vi "DPT Worksheet DOE Audit.vi"(0 "2015?":bool, 1 "Add?":bool, 5 "DOE Data":T1={"Technician"="", "Date"="", "Model"="", "Serial"="", "Total Dry Time(m)"=0.0, "Bone Dry Wt"=0.0, "Initial Wt"=0.0, "Final Wt"=0.0, "Initial Ret"=0.0, "Final Ret"=0.0, "Elect Energy Used"=0.0, "Gas Meter Temp"=0.0, "Gas Meter Pres"=0.0, "Gas Volume"=0.0, "Barometer Temp"=70.0, "Barometer Pres"=0.0, "Gas Corr Fact"=0.0, "Cor Gas Vol"=0.0, "Gas Heat Val"=0.0, "Gas Energy BTU"=0.0, "Gas Energy kwh 4%"=0.0, "Elect Energy kwh 4%"=0.0, "Total  Energy 4%"=0.0, "Gas Vol Init"=0.0, "Gas Vol Fin"=0.0, "Start Time(s)"=0.0, "End Time(s)"=0.0, "Elect Energy Start"=0.0, "Elect Energy End"=0.0, "Per Cycle Efficency"=0.0, "Annual Consumption"=0.0, "Load Cycles"="", "Ambinet Temp"="", "Ambinet RH"="", "Per Cycle Off Mode/Standby Power"=0.0, "Total Energy (Gas + Elect)"=0.0, "Combined Energy Factor"=0.0, "Off Mode Power"=0.0, "Exhaust"="", "Washer Water Temperature ( 60 ± 5°F )"="", "Supply Voltage"="", "Reference Temperature (F)"="", "Reference Pressure (psi)"="", "Standby Power"=0.0}, 12 "Write Form":bool) -> (6 "DOE Data Out":T1={"Technician"="", "Date"="", "Model"="", "Serial"="", "Total Dry Time(m)"=0.0, "Bone Dry Wt"=0.0, "Initial Wt"=0.0, "Final Wt"=0.0, "Initial Ret"=0.0, "Final Ret"=0.0, "Elect Energy Used"=0.0, "Gas Meter Temp"=0.0, "Gas Meter Pres"=0.0, "Gas Volume"=0.0, "Barometer Temp"=70.0, "Barometer Pres"=0.0, "Gas Corr Fact"=0.0, "Cor Gas Vol"=0.0, "Gas Heat Val"=0.0, "Gas Energy BTU"=0.0, "Gas Energy kwh 4%"=0.0, "Elect Energy kwh 4%"=0.0, "Total  Energy 4%"=0.0, "Gas Vol Init"=0.0, "Gas Vol Fin"=0.0, "Start Time(s)"=0.0, "End Time(s)"=0.0, "Elect Energy Start"=0.0, "Elect Energy End"=0.0, "Per Cycle Efficency"=0.0, "Annual Consumption"=0.0, "Load Cycles"="", "Ambinet Temp"="", "Ambinet RH"="", "Per Cycle Off Mode/Standby Power"=0.0, "Total Energy (Gas + Elect)"=0.0, "Combined Energy Factor"=0.0, "Off Mode Power"=0.0, "Exhaust"="", "Washer Water Temperature ( 60 ± 5°F )"="", "Supply Voltage"="", "Reference Temperature (F)"="", "Reference Pressure (psi)"="", "Standby Power"=0.0}, 10 "2015 array":string[][](array[string]), 15 "String":string)   [LabVIEW 2016, in "File Setup.lvlib"]
uses:
  File Setup.lvlib
  Type Definition/DPT Audit Data.ctl
panel:
  # "Add Water Hardness\nand panel"
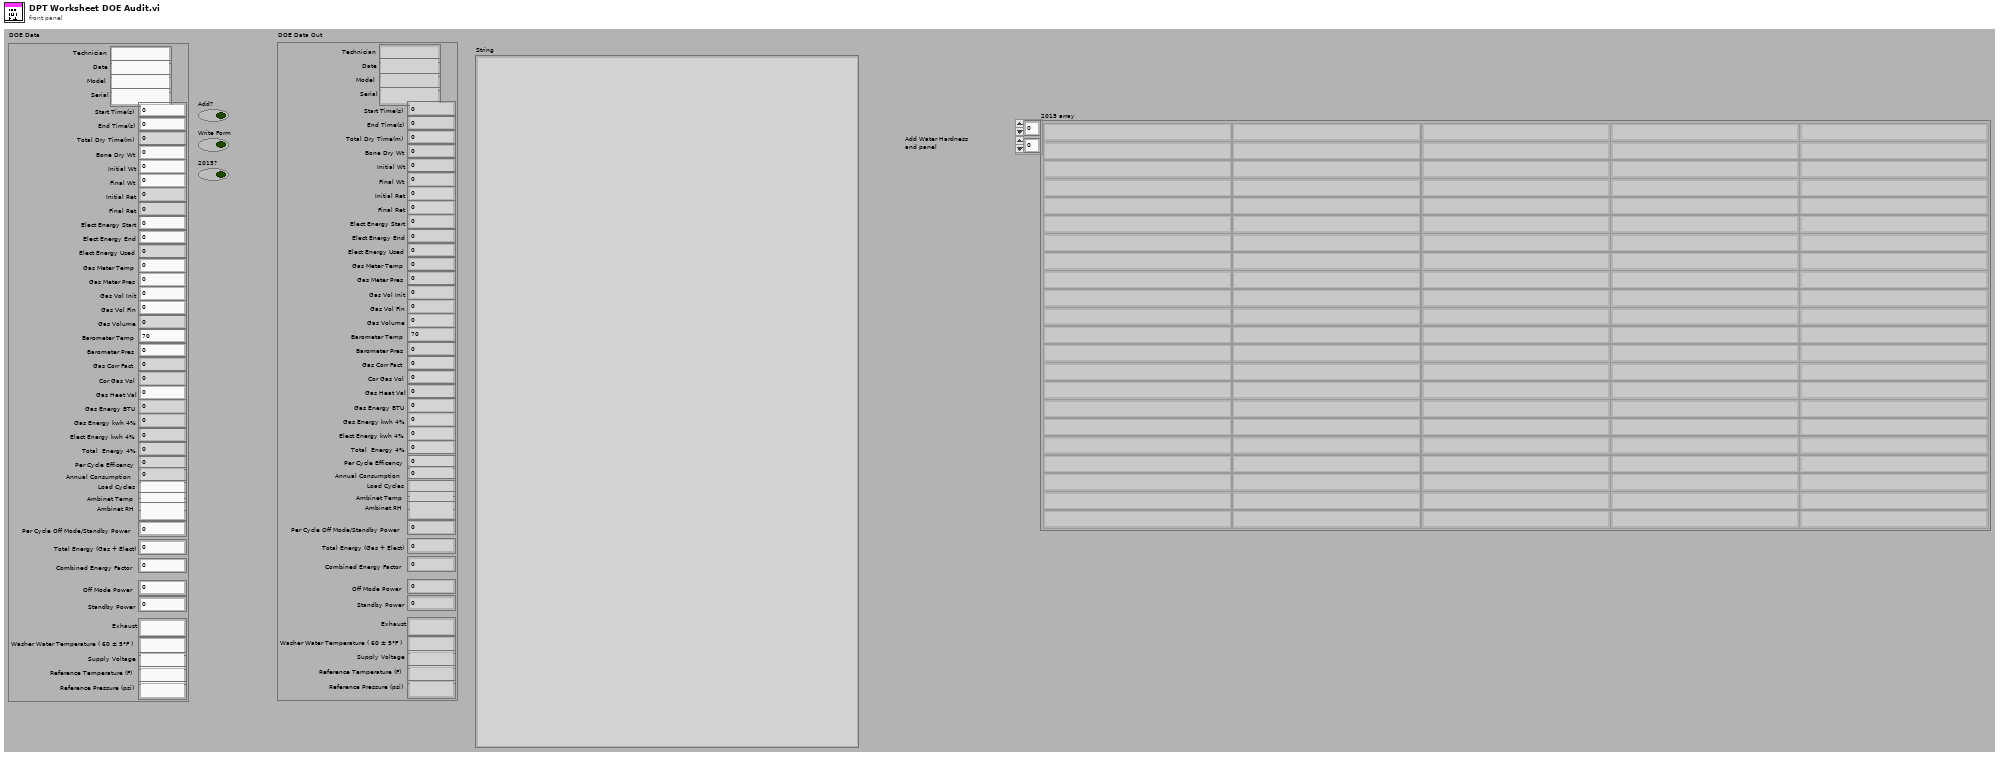
[diagram p1: front panel]
types:
  T1 = typedef "File Setup.lvlib/DPT Audit Data.ctl" = cluster{"Technician":string, "Date":string, "Model":string, "Serial":string, "Total Dry Time(m)":dbl, "Bone Dry Wt":dbl, "Initial Wt":dbl, "Final Wt":dbl, "Initial Ret":dbl, "Final Ret":dbl, "Elect Energy Used":dbl, "Gas Meter Temp":dbl, "Gas Meter Pres":dbl, "Gas Volume":dbl, "Barometer Temp":dbl, "Barometer Pres":dbl, "Gas Corr Fact":dbl, "Cor Gas Vol":dbl, "Gas Heat Val":dbl, "Gas Energy BTU":dbl, "Gas Energy kwh 4%":dbl, "Elect Energy kwh 4%":dbl, "Total  Energy 4%":dbl, "Gas Vol Init":dbl, "Gas Vol Fin":dbl, "Start Time(s)":dbl, "End Time(s)":dbl, "Elect Energy Start":dbl, "Elect Energy End":dbl, "Per Cycle Efficency":dbl, "Annual Consumption":dbl, "Load Cycles":string, "Ambinet Temp":string, "Ambinet RH":string, "Per Cycle Off Mode/Standby Power":dbl, "Total Energy (Gas + Elect)":dbl, "Combined Energy Factor":dbl, "Off Mode Power":dbl, "Exhaust":string, "Washer Water Temperature ( 60 ± 5°F )":string, "Supply Voltage":string, "Reference Temperature (F)":string, "Reference Pressure (psi)":string, "Standby Power":dbl}
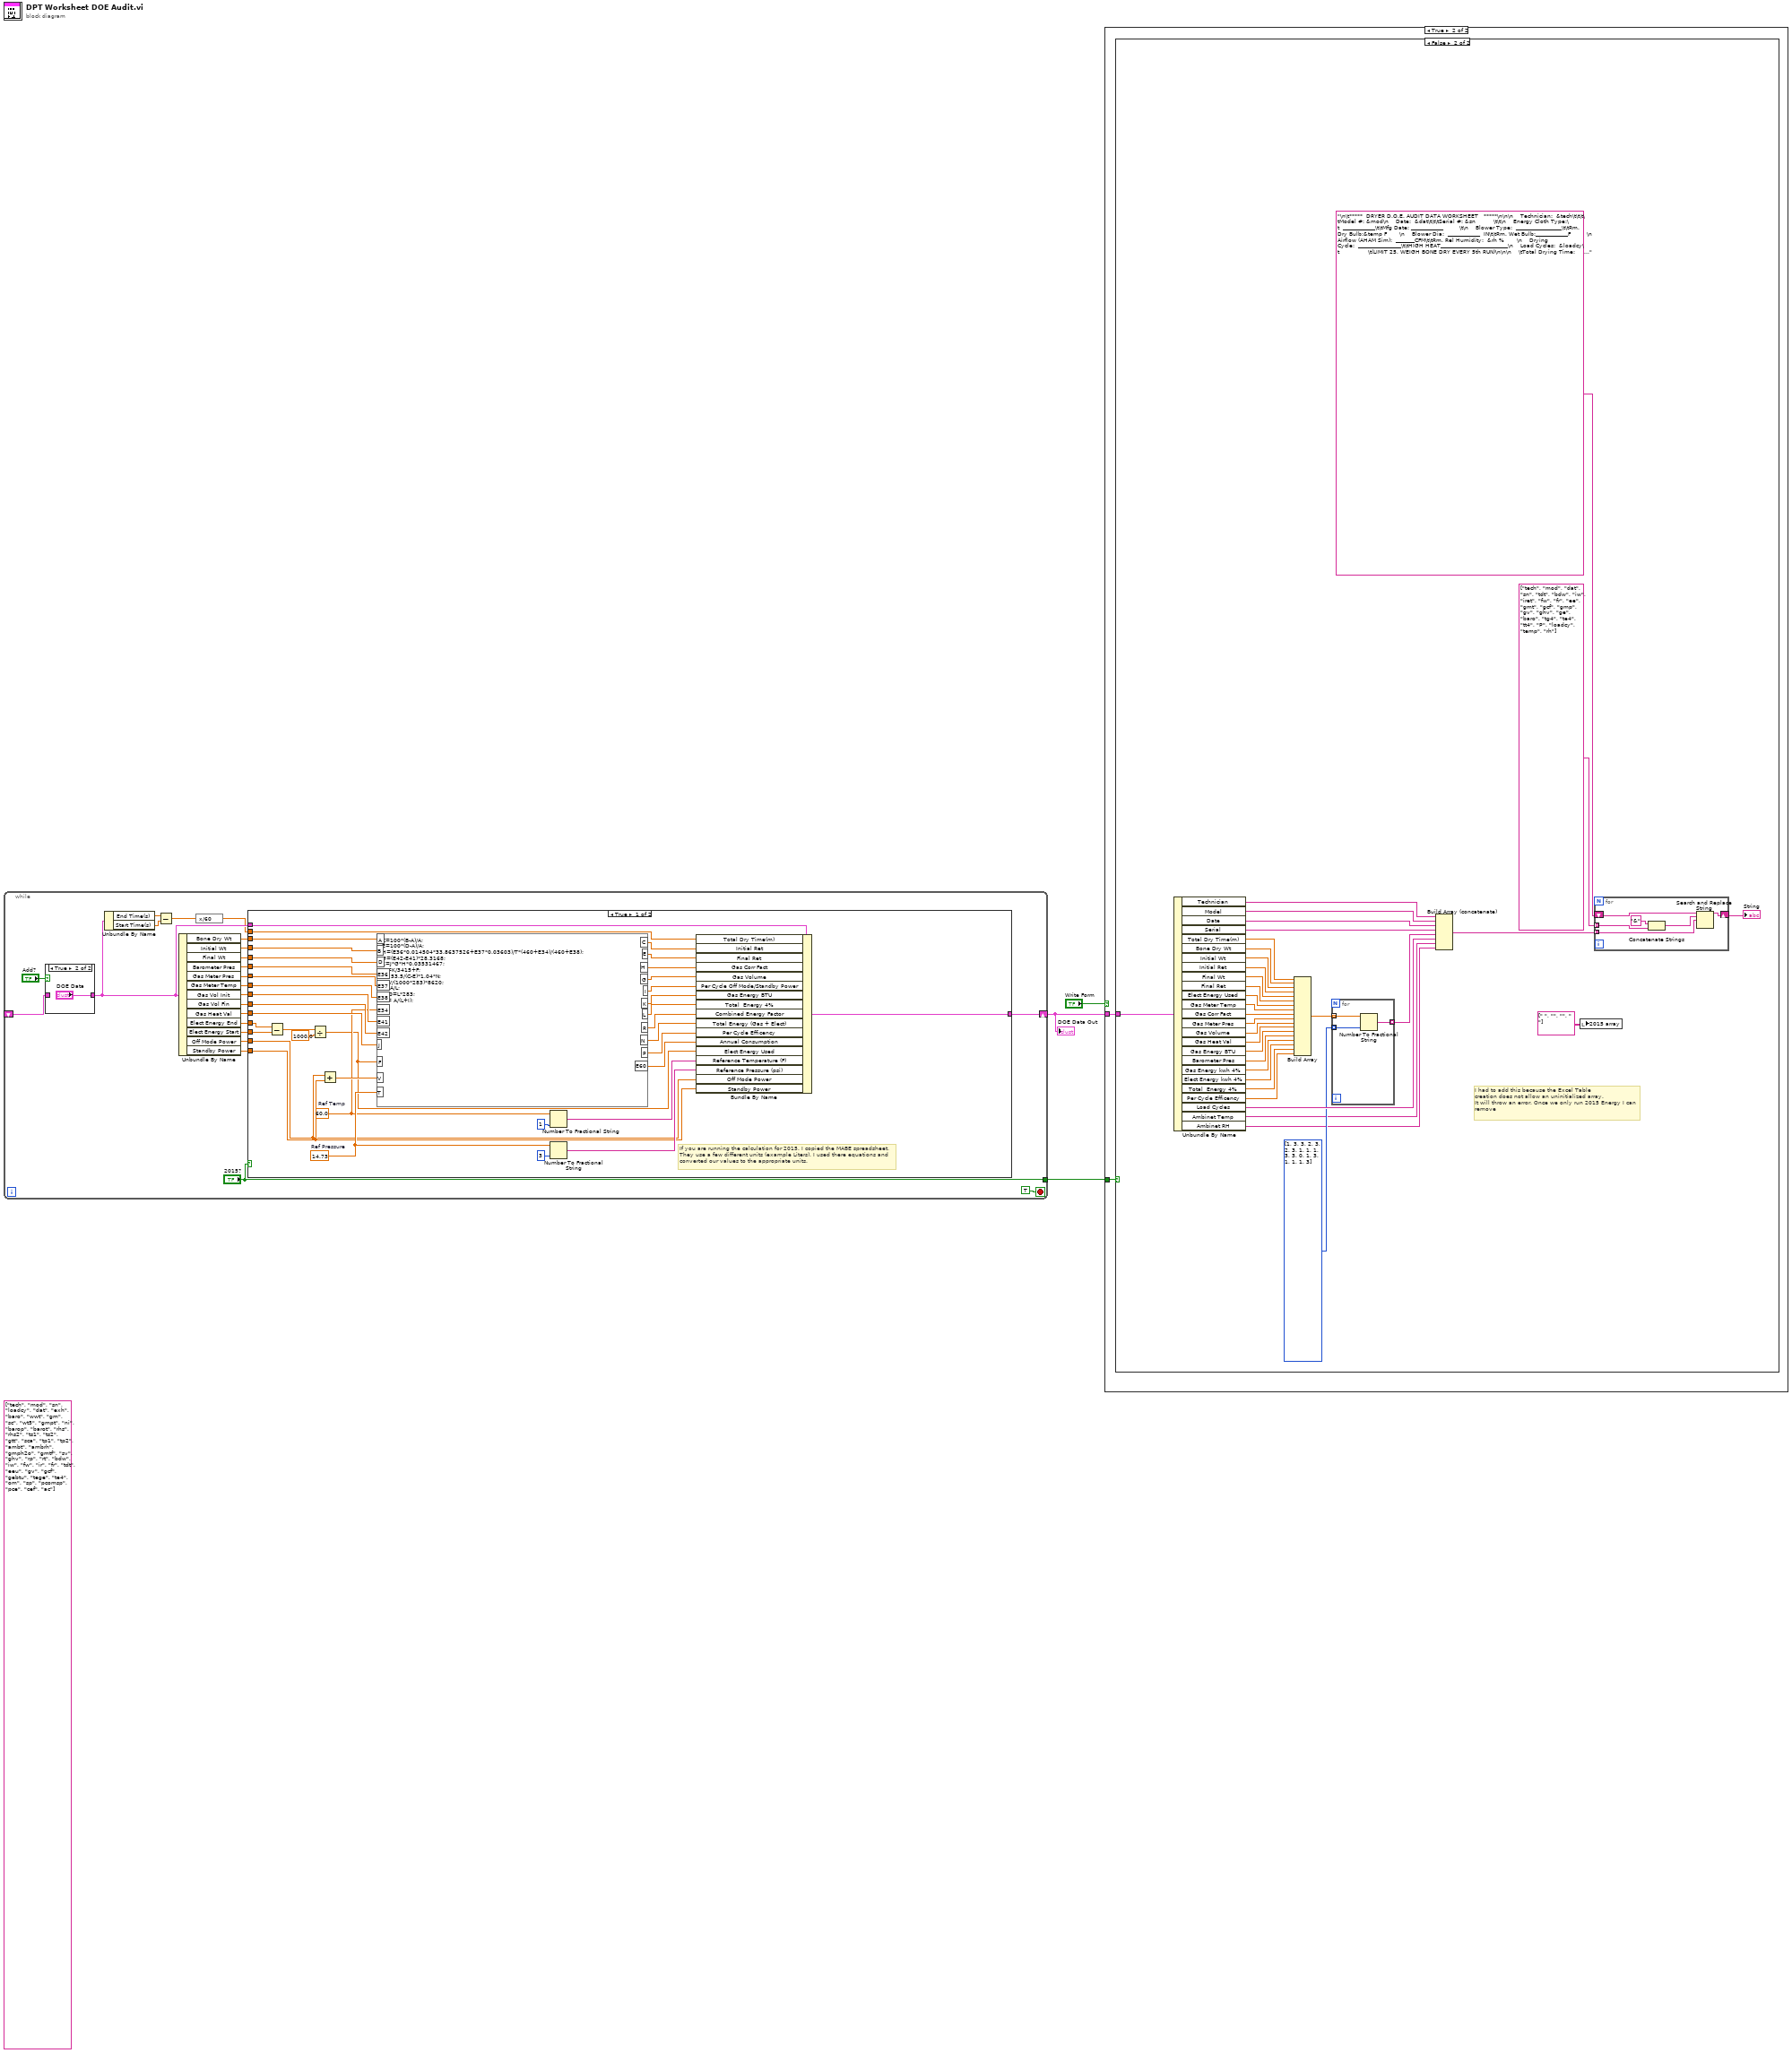
[diagram p0: block diagram]
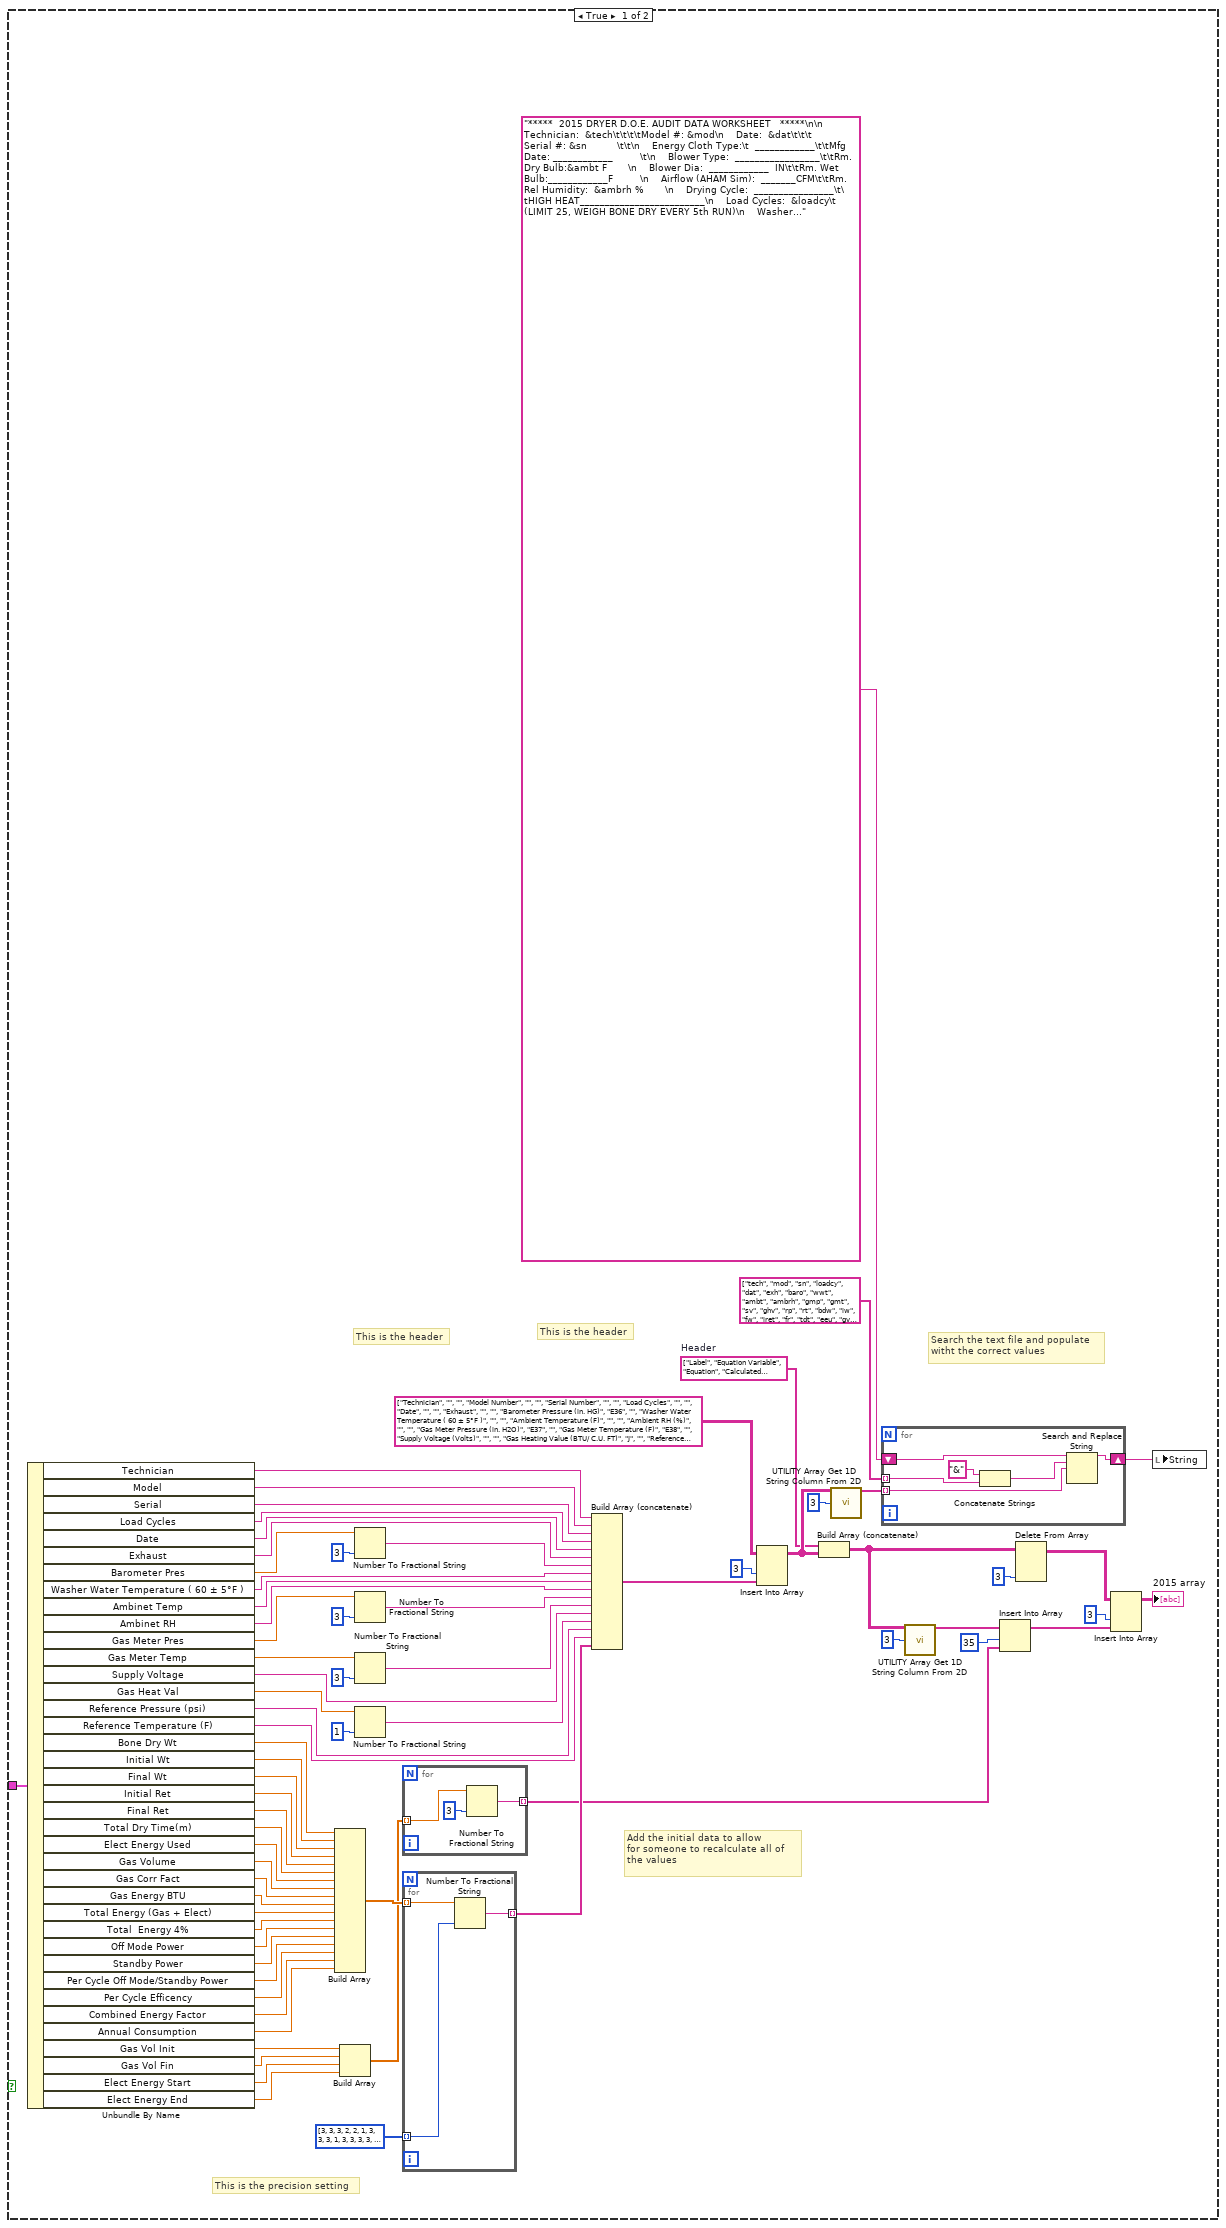
[diagram p3: hidden frame]
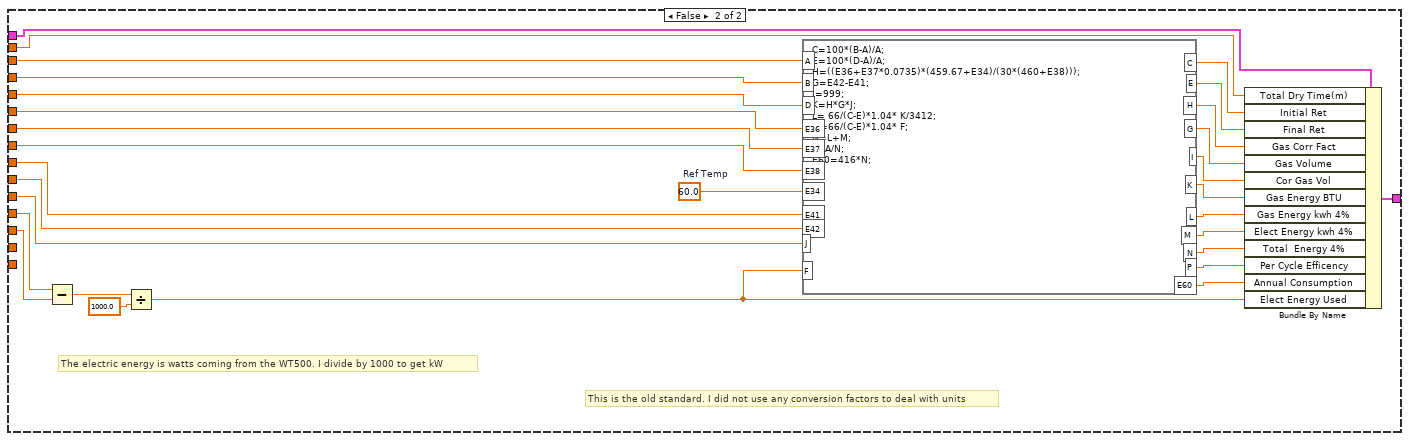
[diagram p4: hidden frame]
diagram:
  (unwired) string[] ["tech", "mod", "sn", "loadcy", "dat", "exh", "baro", "wwt", "gm", "sc", "wt5", "gmpt", "ni", "barop", "barot", "rhs", "rhs2", "ts1", "ts2", "gtt", "sca", "tp1", "tp2", "ambt", "ambrh", "gmph2o", "gmtf", "sv", "ghv", "rp", "rt", "bdw", "iw", "fw", "ir", "fr", "tdt", "eeu", "gv", "gcf", "gebtu", "tege", "te4", "om", "sp", "pcomsp", "pce", "cef", "ac"]
  n1 = while {
    shift-right: [w7] -> w3
    shift-left: _ -> [w25]
    tunnel: ["2015?"] -> w1
    stop <- TRUE stop-if-true
    n2 = case shown="True" "Add?" {
      tunnel: [w93 "DOE Data"] -> w8
      tunnel: w25 -> [w93 _]
      frame False {
      }
      frame True {
      }
    }
    n3 = Unbundle By Name(w8) -> ("End Time(s)"=w23:dbl, "Start Time(s)"=w22:dbl)
    n4 = Subtract(x=w23, y=w22) -> (x-y=w15:dbl)
    n5 = Unbundle By Name(w8) -> ("Bone Dry Wt"=w21:dbl, "Initial Wt"=w20:dbl, "Final Wt"=w19:dbl, "Barometer Pres"=w18:dbl, "Gas Meter Pres"=w17:dbl, "Gas Meter Temp"=w16:dbl, "Gas Vol Init"=w14:dbl, "Gas Vol Fin"=w13:dbl, "Gas Heat Val"=w12:dbl, "Elect Energy End"=w11:dbl, "Elect Energy Start"=w10:dbl, "Off Mode Power"=w9:dbl, "Standby Power"=w4:dbl)
    n6 = expression code="x/60"(w15) -> (w6:dbl)
    n7 = case shown="True" "2015?" {
      tunnel: w21 -> [w63 w92]
      tunnel: w20 -> [w62 w91]
      tunnel: w19 -> [w61 w90]
      tunnel: w18 -> [w60 w88]
      tunnel: w17 -> [w59 w87]
      tunnel: w16 -> [w58 w86]
      tunnel: w14 -> [w57 w85]
      tunnel: w13 -> [w56 w84]
      tunnel: w12 -> [w55 w83]
      tunnel: w11 -> [w54 w82]
      tunnel: w10 -> [w53 w81]
      tunnel: w9 -> [w33 _]
      tunnel: w8 -> [w50 w78]
      tunnel: [w41 w77] -> w7
      tunnel: w6 -> [w49 w76]
      tunnel: w4 -> [w34 _]
      frame True {
        w39 = 14.73  # Ref Pressure
        w30 = 60.0  # Ref Temp
        # "If you are running the calculation for 2015. I copied the MABE spreadsheet.\nThey use a few different units (example Liters). I used there equations and\nconverted our values to the appropriate units."
        n8 = Subtract(x=w54, y=w53) -> (x-y=w52:dbl)
        n9 = Divide(x=w52, y=1000.0) -> (x/y=w28:dbl)
        n10 = Add(x=w33, y=w34) -> (x+y=w31:dbl)
        n11 = formula code="C=100*(B-A)/A;\nE=100*(D-A)/A;\nH=(E36*0.014504*33.8637526+E37*0.03603)/T*(460+E34)/(460+E38);\nG=(E42-E41)*28.3168;\nK=J*G*H*0.03531467;\nN =K/3415+F;\nL= 53.5/(C-E)*1.04*N;\nI=V/(1000*283)*8620;\nP=A/L;\nE60=L*283;\nR = A/(L+I);"("A"=w63, "B"=w62, "D"=w61, "E36"=w60, "E37"=w59, "E34"=w30, "E38"=w58, "E41"=w57, "E42"=w56, "J"=w55, "F"=w28, "V"=w31, "T"=w39) -> ("C"=w48:dbl, "E"=w47:dbl, "H"=w46:dbl, "G"=w45:dbl, "I"=w32:dbl, "K"=w29:dbl, "L"=w44:dbl, "R"=w27:dbl, "N"=w43:dbl, "P"=w42:dbl, "E60"=w37:dbl)
        n12 = Number To Fractional String(number=w30, precision (6)=i16 1) -> (F-format string=w40:string)  [unwired: 2 in]
        n13 = Number To Fractional String(number=w39, precision (6)=i16 3) -> (F-format string=w38:string)  [unwired: 2 in]
        n14 = Bundle By Name(cluster=w50, "Total Dry Time(m)"=w49, "Initial Ret"=w48, "Final Ret"=w47, "Gas Corr Fact"=w46, "Gas Volume"=w45, "Per Cycle Off Mode/Standby Power"=w32, "Gas Energy BTU"=w29, "Total  Energy 4%"=w44, "Combined Energy Factor"=w27, "Total Energy (Gas + Elect)"=w43, "Per Cycle Efficency"=w42, "Annual Consumption"=w37, "Elect Energy Used"=w28, "Reference Temperature (F)"=w40, "Reference Pressure (psi)"=w38, "Off Mode Power"=w33, "Standby Power"=w34) -> (w41:T1)
      }
      frame False {
        w89 = 60.0  # Ref Temp
        # "The electric energy is watts coming from the WT500. I divide by 1000 to get kW"
        # "This is the old standard. I did not use any conversion factors to deal with units"
        n15 = Subtract(x=w82, y=w81) -> (x-y=w80:dbl)
        n16 = Divide(x=w80, y=1000.0) -> (x/y=w64:dbl)
        n17 = formula code="C=100*(B-A)/A;\nE=100*(D-A)/A;\nH=((E36+E37*0.0735)*(459.67+E34)/(30*(460+E38)));\nG=E42-E41;\nI=999;\nK=H*G*J;\nL= 66/(C-E)*1.04* K/3412;\nM=66/(C-E)*1.04* F;\nN=L+M;\nP=A/N;\nE60=416*N;"("A"=w92, "B"=w91, "D"=w90, "E36"=w88, "E37"=w87, "E34"=w89, "E38"=w86, "E41"=w85, "E42"=w84, "J"=w83, "F"=w64) -> ("C"=w75:dbl, "E"=w74:dbl, "H"=w73:dbl, "G"=w72:dbl, "I"=w71:dbl, "K"=w70:dbl, "L"=w69:dbl, "M"=w68:dbl, "N"=w67:dbl, "P"=w66:dbl, "E60"=w65:dbl)
        n18 = Bundle By Name(cluster=w78, "Total Dry Time(m)"=w76, "Initial Ret"=w75, "Final Ret"=w74, "Gas Corr Fact"=w73, "Gas Volume"=w72, "Cor Gas Vol"=w71, "Gas Energy BTU"=w70, "Gas Energy kwh 4%"=w69, "Elect Energy kwh 4%"=w68, "Total  Energy 4%"=w67, "Per Cycle Efficency"=w66, "Annual Consumption"=w65, "Elect Energy Used"=w64) -> (w77:T1)
      }
    }
  }
  "DOE Data Out" <- w3
  n19 = case shown="True" "Write Form" {
    tunnel: w3 -> [_ w96]
    tunnel: w1 -> [_ w95]
    frame False {
    }
    frame True {
      n20 = case shown="False" w95 {
        tunnel: w96 -> [w164 w213]
        frame True {
          w112 = string[] ["Label", "Equation Variable", "Equation", "Calculated Result"]  # Header
          # "Search the text file and populate \nwitht the correct values"
          # "This is the header"
          # "This is the header"
          # "Add the initial data to allow\nfor someone to recalculate all of \nthe values"
          # "This is the precision setting"
          n21 = Unbundle By Name(w164) -> ("Technician"=w163:string, "Model"=w162:string, "Serial"=w161:string, "Load Cycles"=w160:string, "Date"=w159:string, "Exhaust"=w158:string, "Barometer Pres"=w157:dbl, "Washer Water Temperature ( 60 ± 5°F )"=w155:string, "Ambinet Temp"=w154:string, "Ambinet RH"=w153:string, "Gas Meter Pres"=w152:dbl, "Gas Meter Temp"=w150:dbl, "Supply Voltage"=w148:string, "Gas Heat Val"=w147:dbl, "Reference Pressure (psi)"=w145:string, "Reference Temperature (F)"=w144:string, "Bone Dry Wt"=w143:dbl, "Initial Wt"=w142:dbl, "Final Wt"=w141:dbl, "Initial Ret"=w140:dbl, "Final Ret"=w139:dbl, "Total Dry Time(m)"=w138:dbl, "Elect Energy Used"=w137:dbl, "Gas Volume"=w136:dbl, "Gas Corr Fact"=w135:dbl, "Gas Energy BTU"=w134:dbl, "Total Energy (Gas + Elect)"=w133:dbl, "Total  Energy 4%"=w132:dbl, "Off Mode Power"=w131:dbl, "Standby Power"=w119:dbl, "Per Cycle Off Mode/Standby Power"=w130:dbl, "Per Cycle Efficency"=w129:dbl, "Combined Energy Factor"=w128:dbl, "Annual Consumption"=w127:dbl, "Gas Vol Init"=w111:dbl, "Gas Vol Fin"=w110:dbl, "Elect Energy Start"=w109:dbl, "Elect Energy End"=w108:dbl)
          n22 = Build Array(w143, w142, w141, w140, w139, w138, w137, w136, w135, w134, w133, w132, w131, w119, w130, w129, w128, w127) -> (w167:dbl[])
          n23 = Build Array(w111, w110, w109, w108) -> (w107:dbl[])
          n24 = Number To Fractional String(number=w157, precision (6)=i16 3) -> (F-format string=w156:string)  [unwired: 2 in]
          n25 = Number To Fractional String(number=w152, precision (6)=i16 3) -> (F-format string=w151:string)  [unwired: 2 in]
          n26 = Number To Fractional String(number=w150, precision (6)=i16 3) -> (F-format string=w149:string)  [unwired: 2 in]
          n27 = Number To Fractional String(number=w147, precision (6)=i16 1) -> (F-format string=w146:string)  [unwired: 2 in]
          n28 = for {
            tunnel: w107 -> [w169] mode=indexing
            tunnel: [w170] -> w103 mode=indexing
            n29 = Number To Fractional String(number=w169, precision (6)=i16 3) -> (F-format string=w170:string)  [unwired: 2 in]
          }
          n30 = for {
            tunnel: w167 -> [w177] mode=indexing
            tunnel: [w179] -> w166 mode=indexing
            tunnel: i16[] [3, 3, 3, 2, 2, 1, 3, 3, 3, 1, 3, 3, 3, 3, 2, 3, 3, 0, 0] -> [w178] mode=indexing
            n31 = Number To Fractional String(number=w177, precision (6)=w178) -> (F-format string=w179:string)  [unwired: 2 in]
          }
          n32 = Build Array (concatenate)(w163, w162, w161, w160, w159, w158, w156, w155, w154, w153, w151, w149, w148, w146, w145, w144, w166) -> (w124:string[])
          n33 = Insert Into Array(array=string[][] [["Technician", "", ""], ["Model Number", "", ""], ["Serial Number", "", ""], ["Load Cycles", "", ""], ["Date", "", ""], ["Exhaust", "", ""], ["Barometer Pressure (in. HG)", "E36", ""], ["Washer Water Temperature ( 60 ± 5°F )", "", ""], ["Ambient Temperature (F)", "", ""], ["Ambient RH (%)", "", ""], ["Gas Meter Pressure (in. H2O)", "E37", ""], ["Gas Meter Temperature (F)", "E38", ""], ["Supply Voltage (Volts)", "", ""], ["Gas Heating Value (BTU/ C.U. FT)", "J", ""], ["Reference Pressure (PSI)", "T", ""], ["Reference Temperature (F)", "E34", ""], ["Bone Dry Weight (lbs)", "A", ""], ["Initial Weight (lbs)", "B", ""], ["Final Weight (lbs)", "D", ""], ["Initial Humidity (%)", "C", "C=100*(B-A)/A"], ["Final Humidity (%)", "E", "E=100*(D-A)/A"], ["Total Dry Time (Minutes)", "", ""], ["Electric Energy Used (kWh)", "F", ""], ["Gas Volume (Liters)", "G", "G=(E42-E41)*28.3168"], ["Gas Volume Correction Factor", "H", "H=(E36*0.014504*33.8637526+E37*0.03603)/T*(460+E34)/(460+E38)"], ["Gas Energy Consumption (BTU)", "K", "K=J*G*H*0.03531467"], ["Total Energy (Gas + Electric) (kWh)", "N", "N =K/3415+F"], ["Electric Energy Corrected (kWh)", "L", "L= 53.5/(C-E)*1.04*N"], ["Off Mode (Watts)", "", ""], ["Standby Mode (Watts)", "", "I=V/(1000*283)*8620"], ["Per-Cycle Standby and Off Modes Energy Consumption (kWh)", "I", "P=A/L"], ["Energy Factor (lb/kWh)", "P", "R = A/(L+I)"], ["Combined Energy Factor (lbs/kWh)", "R", "E60=L*283"], ["Annual Energy Consumption (kWh/Year)", "E60", ""], ["Gas Volume Initial (CU.FT)", "", ""], ["Gas Volume Final (CU.FT)", "", ""], ["Electric Energy Start (Watt Hours)", "", ""], ["Electric Energy End (Watt Hours)", "", ""]], index (col)=3 ("disabled index (col)"), new element=w124) -> (w113:string[][])  [unwired: 1 in]
          n34 = Build Array (concatenate)(w112, w113) -> (w102:string[][])
          n35 = call "UTILITY Array Get 1D String Column From 2D.vi"("2D Array Data"=w113, "column index"=3) -> ("Column Data"=w114:string[])  [unwired: 13 in]
          n36 = for {
            tunnel: string[] ["tech", "mod", "sn", "loadcy", "dat", "exh", "baro", "wwt", "ambt", "ambrh", "gmp", "gmt", "sv", "ghv", "rp", "rt", "bdw", "iw", "fw", "iret", "fr", "tdt", "eeu", "gv", "gcf", "gebtu", "tege", "te4", "om", "sp", "pcomsp", "P", "cef", "ac"] -> [w175] mode=indexing
            tunnel: w114 -> [w172] mode=indexing
            shift-right: [w171] -> w116
            shift-left: "*****  2015 DRYER D.O.E. AUDIT DATA WORKSHEET   *****\n\n    Technician:  &tech\t\t\t\tModel #: &mod\n    Date:  &dat\t\t\t                Serial #: &sn          \t\t\n    Energy Cloth Type:\t  ____________\t\tMfg Date: ____________         \t\n    Blower Type:  _________________\t\tRm. Dry Bulb:&ambt F       \n    Blower Dia:  ____________  IN\t\tRm. Wet Bulb:____________F         \n    Airflow (AHAM Sim):  _______CFM\t\tRm. Rel Humidity:  &ambrh %       \n    Drying Cycle:  ________________\t\tHIGH HEAT_________________________\n    Load Cycles:  &loadcy\t                (LIMIT 25, WEIGH BONE DRY EVERY 5th RUN)\n    Washer Water Temperature ( 60 ± 5°F ): &wwt\n    Exhaust Type: &exh\n    Equipment Calibration: Reference Spreadsheet File\n\n    \tTotal Drying Time:     &tdt  min\n(A) \tBone Dry Weight:       &bdw lb\t\t\t(ALL WEIGHTS FROM REF SCALE)\n(B) \tInitial Wt. Wet Load:  &iw  lb\t\t(C) Initial Ret. 100*(B-A)/A:  &iret %\n(D) \tFinal Wt. Dried Load:  &fw  lb\t\t(E) Final Ret.   100*(D-A)/A:  &fr %\n\nELECTRICAL ENERGY:\n\n(F) Electrical Energy Used:  &eeu  kwh\n\nGAS ENERGY:\n\n\tGas Meter Temp:   &gmt F\t   (H) Gas Corr. Factor:     &gcf  ++ \n\tGas Meter Press:  &gmp in H20      (J) Gas Heating Value:    &ghv  BTU/CUFT           \n(G) Metered Gas Vol:      &gv Liters (K) Gas Energy (G*H*J*0.0353):     &gebtu BTU\t     \n           \nBarometer Press:  &baro in HG\t           Supply Voltage: &sv\t\n\nReference Pressure: &rp                    Reference Temperature: &rt\n\n++ From PC program per US Bureau of Stds, C417,1938\n \n(N) Total Energy (Gas + Electric) (kWh): &tege\n    [(K/3415)+F]\n\n(L) Per cycle Total Electric Energy Consumption adjusted to 4%:  &te4 KWH/CYCLE\n    ([53.5/(C-E)]*1.04*N)\n\n(I) Per Cycle Off Mode/Standby Mode Power: &pcomsp\n    [V/(1000*283)*8620] \n\n(V) Standby Mode Power: &sp Watts\n    Off Mode Power: &om Watts \n         Off Mode > 0 & Standby Mode > 0: [0.5*(Off Mode+Standby Mode)]\n         Off Mode > 0 & Standby Mode = 0: [(Off Mode+Standby Mode)]\n\n(E60) Annual Consumption: [(L*283)]  &ac kwh\n\n(R) Combined Energy Factor: [A/(L+I)] &cef\n\n***********************************************************\n   * (P) Per Cycle Energy Efficiency (A/L): &P\n***********************************************************" -> [w176]
            n37 = Concatenate Strings("&" ("string"), w175) -> (w173:string)
            n38 = Search and Replace String(input string=w176, search string=w173, replace string=w172) -> (result string=w171:string)  [unwired: 5 in, 3 out]
          }
          n39 = call "UTILITY Array Get 1D String Column From 2D.vi"("2D Array Data"=w102, "column index"=3) -> ("Column Data"=w105:string[])  [unwired: 13 in]
          n40 = Insert Into Array(array=w105, index=35 ("index (row)"), new element=w103) -> (w99:string[])
          n41 = Delete From Array(array=w102, index (col)=3 ("column index")) -> (array with subset deleted=w100:string[][])  [unwired: 2 in, 1 out]
          n42 = Insert Into Array(array=w100, index (col)=3 ("disabled index (col)"), new element=w99) -> (→"2015 array":string[][])  [unwired: 1 in]
          n43 = local write "String"(w116) -> ()
        }
        frame False {
          # "I had to add this because the Excel Table \ncreation does not allow an uninitialized array.\nIt will throw an error. Once we only run 2015 Energy I can\nremove"
          n44 = Unbundle By Name(w213) -> ("Technician"=w190:string, "Model"=w191:string, "Date"=w192:string, "Serial"=w193:string, "Total Dry Time(m)"=w212:dbl, "Bone Dry Wt"=w211:dbl, "Initial Wt"=w210:dbl, "Initial Ret"=w209:dbl, "Final Wt"=w208:dbl, "Final Ret"=w207:dbl, "Elect Energy Used"=w206:dbl, "Gas Meter Temp"=w205:dbl, "Gas Corr Fact"=w204:dbl, "Gas Meter Pres"=w203:dbl, "Gas Volume"=w202:dbl, "Gas Heat Val"=w201:dbl, "Gas Energy BTU"=w200:dbl, "Barometer Pres"=w199:dbl, "Gas Energy kwh 4%"=w198:dbl, "Elect Energy kwh 4%"=w197:dbl, "Total  Energy 4%"=w182:dbl, "Per Cycle Efficency"=w196:dbl, "Load Cycles"=w187:string, "Ambinet Temp"=w185:string, "Ambinet RH"=w184:string)
          n45 = Build Array(w212, w211, w210, w209, w208, w207, w206, w205, w204, w203, w202, w201, w200, w199, w198, w197, w182, w196) -> (w195:dbl[])
          n46 = for {
            tunnel: w195 -> [w216] mode=indexing
            tunnel: [w215] -> w194 mode=indexing
            tunnel: i16[] [1, 3, 3, 2, 3, 2, 3, 1, 1, 1, 3, 3, 0, 1, 3, 1, 1, 1, 3] -> [w214] mode=indexing
            n47 = Number To Fractional String(number=w216, precision (6)=w214) -> (F-format string=w215:string)  [unwired: 2 in]
          }
          n48 = Build Array (concatenate)(w190, w191, w192, w193, w194, w187, w185, w184) -> (w188:string[])
          n49 = local write "2015 array"(string[][] [[" ", ""], ["", " "]]) -> ()
          n50 = for {
            tunnel: string[] ["tech", "mod", "dat", "sn", "tdt", "bdw", "iw", "iret", "fw", "fr", "ee", "gmt", "gcf", "gmp", "gv", "ghv", "ge", "baro", "tg4", "te4", "tt4", "P", "loadcy", "temp", "rh"] -> [w221] mode=indexing
            tunnel: w188 -> [w218] mode=indexing
            shift-right: [w217] -> w181
            shift-left: "\n\t*****  DRYER D.O.E. AUDIT DATA WORKSHEET   *****\n\n\n    Technician:  &tech\t\t\t\tModel #: &mod\n    Date:  &dat\t\t\tSerial #: &sn          \t\t\n    Energy Cloth Type:\t  ____________\t\tMfg Date: ____________         \t\n    Blower Type:  _________________\t\tRm. Dry Bulb:&temp F       \n    Blower Dia:  ____________  IN\t\tRm. Wet Bulb:____________F         \n    Airflow (AHAM Sim):  _______CFM\t\tRm. Rel Humidity:  &rh %       \n    Drying Cycle:  ________________\t\tHIGH HEAT_________________________\n    Load Cycles:  &loadcy\t                \t(LIMIT 25, WEIGH BONE DRY EVERY 5th RUN)\n\n\n    \tTotal Drying Time:     &tdt  min\n(A) \tBone Dry Weight:       &bdw lb\t\t\t(ALL WEIGHTS FROM REF SCALE)\n(B) \tInitial Wt. Wet Load:  &iw  lb\t\t(C) Initial Ret. [(B-A)/A]:  &iret %\n(D) \tFinal Wt. Dried Load:  &fw  lb\t\t(E) Final Ret.   [(D-A)/A]:  &fr %\n\nELECTRICAL ENERGY:\n\n(F) Electrical Energy Used:  &ee  kwh\n\nGAS ENERGY:\n\n\tGas Meter Temp:   &gmt F\t        \t(H) Gas Corr. Factor:     &gcf  ++ \n\tGas Meter Press:  &gmp in H20           \n(G) Metered Gas Vol:      &gv CU FT\t\t(J) Gas Heating Value:    &ghv  BTU/CUFT\n\t                                        (K) Gas Energy (G*H*J):     &ge BTU\n\tBarometer Press:  &baro in HG\t\t\n\n++ From PC program per US Bureau of Stds, C417,1938 \n\n(M) Per cycle Total Electric Energy Consumption adjusted to 4%:  &te4 KWH/CYCLE\n([66/(C-E)]*1.04*F)\n\n(N) Per cycle Total Gas Energy Consumption adjusted to 4%:  &tg4 KWH/CYCLE\n([66/(C-E)]*1.04*K)/3412\n\n(O) Total Energy Used in kwh (M+N):  &tt4 kwh\n***********************************************************\n   * (P) Per Cycle Energy Efficiency (A/O): &P\n***********************************************************\n" -> [w222]
            n51 = Concatenate Strings("&" ("string"), w221) -> (w219:string)
            n52 = Search and Replace String(input string=w222, search string=w219, replace string=w218) -> (result string=w217:string)  [unwired: 5 in, 3 out]
          }
          "String" <- w181
        }
      }
    }
  }
